vi "DequeueSub.vi"(7 "nonEmpty":refnum<k4>, 8 "element in":T1, 11 "SubChannel in":refnum<class "SubChannelCPU.lvclass">) -> (0 "element out":T1, 1 "count":i32, 2 "wait":bool, 3 "SubChannel out":refnum<class "SubChannelCPU.lvclass">, 4 "last element?":bool, 5 "valid?":bool)   [LabVIEW 2019, in "MessengerM.lvlib" / "SubChannelCPU.lvclass"]
uses:
  SubChannelCPU.lvclass
  <resource>/ChannelSupport/_ChannelSupport/PipeLogic2/PipeLogic2.lvclass
  Element.ctl
  MessengerM.lvlib
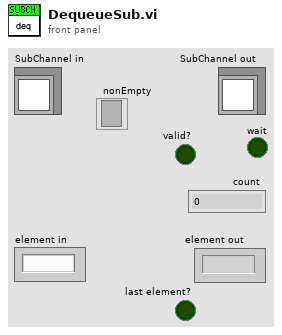
[diagram p1: front panel]
types:
  T1 = typedef "MessengerM.lvlib/Element.ctl" = string
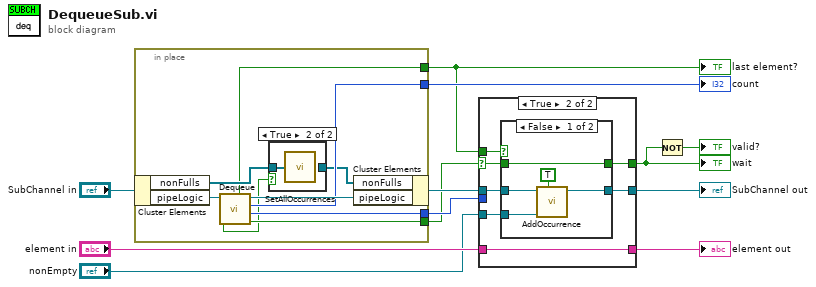
[diagram p0: block diagram]
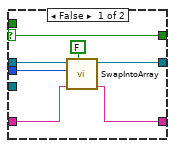
[diagram p3: hidden frame]
diagram:
  n1 = in-place {
    in-place-border: [w20] -> w6
    in-place-border: [w18] -> w9
    in-place-border: [w17] -> w8
    in-place-border: [w13] -> w3
    n2 = in-place-cluster #1("SubChannel in") -> ("nonFulls"=w16:refnum<k4>[], "pipeLogic"=w19:refnum<class "PipeLogic2.lvclass">)
    n3 = call <resource>:"Dequeue.vi"("pipeLogic in"=w19) -> ("wait"=w20:bool, "index"=w17:i32, "count"=w18:i32, "pipeLogic out"=w21:refnum<class "PipeLogic2.lvclass">, "last element out"=w13:bool, "set nonfull"=w15:bool)  [unwired: 5 in]
    n4 = case shown="True" w15 {
      tunnel: w16 -> [w22 w23]
      tunnel: [w22 _] -> w14
      frame False {
      }
      frame True {
        n5 = call "SetAllOccurrences.vi"("occurrences"=w23) -> ()
      }
    }
    n6 = in-place-cluster #1("nonFulls"=w14, "pipeLogic"=w21) -> (w12:refnum<class "SubChannelCPU.lvclass">)
  }
  "count" <- w9
  "last element?" <- w3
  n7 = case shown="True" w6 {
    selector: w6 -> [w24 w31]
    tunnel: [w29 w35] -> w4
    tunnel: w12 -> [w30 w36]
    tunnel: "element in" -> [w28 w37]
    tunnel: [w27 w37] -> w10
    tunnel: w8 -> [w26 _]
    tunnel: "nonEmpty" -> [_ w34]
    tunnel: [w24 w32] -> w2
    tunnel: w3 -> [_ w33]
    frame False {
      n8 = call "SwapIntoArray.vi"("enq"=FALSE, "element in"=w28, "index"=w26, "SubChannel in"=w30) -> ("element out"=w27:T1, "SubChannel out"=w29:refnum<class "SubChannelCPU.lvclass">)  [unwired: 5 in, 1 out]
    }
    frame True {
      n9 = case shown="False" w33 {
        tunnel: w36 -> [w42 w43]
        tunnel: [w41 w43] -> w35
        tunnel: w34 -> [w39 _]
        tunnel: [w38 _] -> w32
        tunnel: w31 -> [w38 _]
        frame False {
          n10 = call "AddOccurrence.vi"("nonEmpty"=TRUE, "occ"=w39, "SubChannel in"=w42) -> ("SubChannel out"=w41:refnum<class "SubChannelCPU.lvclass">)  [unwired: 8 in]
        }
        frame True {
          # "don't wait if\nlast elt -->\nelt not valid"
        }
      }
    }
  }
  "SubChannel out" <- w4
  "element out" <- w10
  "wait" <- w2
  n11 = Not(x=w2) -> (.not. x?=→"valid?":bool)
